vi "Frequency Response Function (Mag-Phase) 1-N.vi"(0 "time signal X":waveform(dbl), 1 "restart averaging (F)":bool, 2 "window parameter":dbl=nan, 5 "time signals Y":waveform(dbl)[](array[waveform]), 7 "window":T1=1 items=["Rectangle"=0, "Hanning"=1, "Hamming"=2, "Blackman-Harris"=3, "Exact Blackman"=4, "Blackman"=5, "Flat Top"=6, "4 Term B-Harris "=7, "7 Term B-Harris"=8, "Low Sidelobe"=9, "Blackman Nuttall"=11, "Triangle"=30, "Bartlett-Hanning"=31, "Bohman"=32, "Parzen"=33, "Welch"=34, "Kaiser"=60, "Dolph-Chebyshev"=61, "Gaussian"=62], 9 "view":T3, 11 "error in (no error)":errorcluster, 12 "averaging parameters":T2={"averaging mode"=enum."No averaging", "weighting mode"=enum."Exponential", "number of averages"=10} {"number of averages" min=1}, 13 "FRF Mode":enum16{"H1", "H2", "H3"}(ring)) -> (3 "averaging done":bool, 4 "magnitudes":cluster{"f0":dbl, "df":dbl, "magnitude":dbl[]}[](array[cluster]) {"magnitude" format="%.2p"; "f0" format="%0.2p"; "df" format="%0.2p"}, 6 "phases":cluster{"f0":dbl, "df":dbl, "phase":dbl[]}[](array[cluster]) {"phase" format="%.2p"; "f0" format="%0.2p"; "df" format="%0.2p"}, 8 "coherences":cluster{"f0":dbl, "df":dbl, "coherence":dbl[]}[](array[cluster]), 10 "averages completed":dbl format="%.2p", 15 "error out":errorcluster)   [LabVIEW 2020, in "NI_MAPro.lvlib"]
doc: "Computes the frequency response and the coherence based on the input signals. Results are returned as <B>magnitude</B>, <B>phase</B>, and <B>coherence</B>."
uses:
  NI_MAPro.lvlib
  windowTd.ctl
  2-chan State.ctl
  NI_MABase.lvlib
  NI_AALPro.lvlib
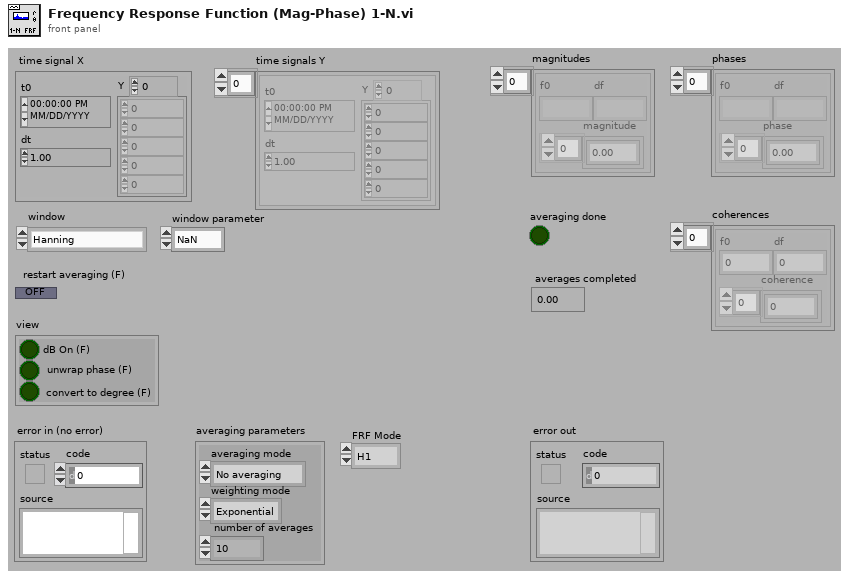
[diagram p1: front panel]
types:
  T1 = typedef "NI_AALPro.lvlib/windowTd.ctl" = u32
  T2 = cluster{"averaging mode":enum16{"No averaging", "Vector averaging", "RMS averaging", "Peak hold"}, "weighting mode":enum16{"Linear", "Exponential"}, "number of averages":u32}
  T3 = cluster{"dB On (F)":bool, "unwrap phase (F)":bool, "convert to degree (F)":bool}
  T4 = typedef "NI_MAPro.lvlib/2-chan State.ctl" = cluster{"Sx":cdb[], "Sy":cdb[], "Sxx":dbl[], "Syy":dbl[], "Sxy":cdb[], "block size":i32, "df":dbl, "dt":dbl, "avgs completed":dbl, "spectrum parameters":cluster{"averaging parameters":cluster{"averaging mode":enum16{"No averaging", "Vector averaging", "RMS averaging", "Peak hold"}, "weighting mode":enum16{"Linear", "Exponential"}, "number of averages":u32}, "window":T1}, "lin avg done":bool, "t0 history":dbl, "dt history":dbl, "timestamp":dbl}
  T5 = cluster{"f0":dbl, "df":dbl, "imag or phase":dbl[]}
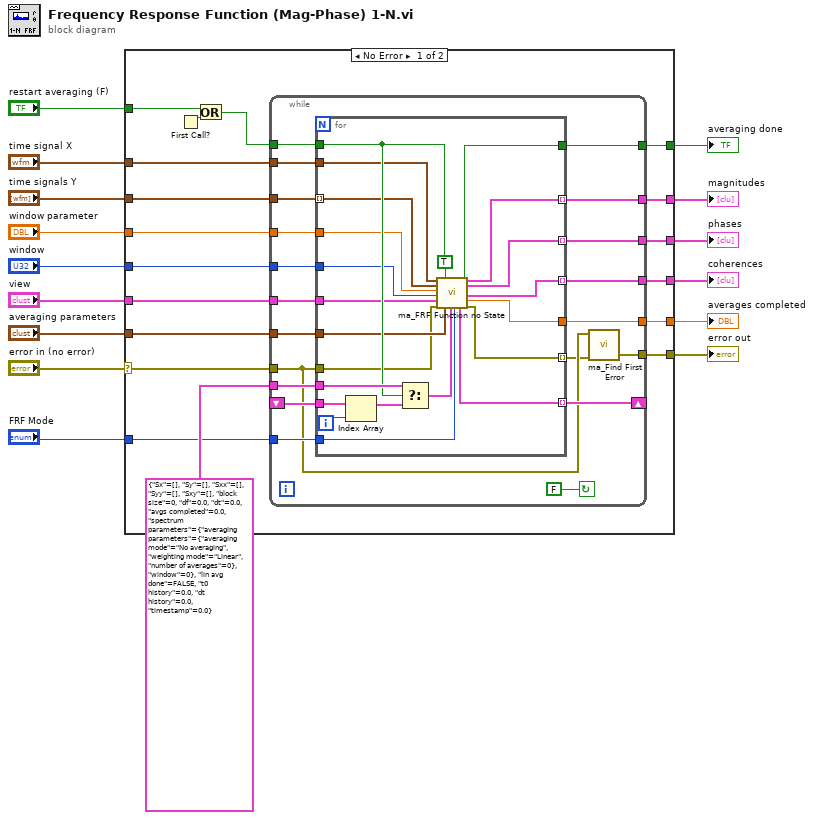
[diagram p0: block diagram]
diagram:
  n1 = case shown="No Error" "error in (no error)" {
    selector: "error in (no error)" -> [w30 w76]
    tunnel: [w29 w76] -> w14
    tunnel: "FRF Mode" -> [w28 _]
    tunnel: "averaging parameters" -> [w27 _]
    tunnel: "view" -> [w26 _]
    tunnel: "window" -> [w25 _]
    tunnel: "time signals Y" -> [w24 _]
    tunnel: "time signal X" -> [w23 _]
    tunnel: "restart averaging (F)" -> [w22 _]
    tunnel: "window parameter" -> [w21 _]
    tunnel: [w20 _] -> w5
    tunnel: [w19 _] -> w4
    tunnel: [w18 _] -> w3
    tunnel: [w17 _] -> w2
    tunnel: [w16 _] -> w1
    frame No Error {
      n2 = First Call?() -> (First Call?: T/F=w33:bool)
      n3 = Or(x=w22, y=w33) -> (x .or. y?=w31:bool)
      n4 = while {
        tunnel: T4 {"Sx"=[], "Sy"=[], "Sxx"=[], "Syy"=[], "Sxy"=[], "block size"=0, "df"=0.0, "dt"=0.0, "avgs completed"=0.0, "spectrum parameters"={"averaging parameters"={"averaging mode"=enum."No averaging", "weighting mode"=enum."Linear", "number of averages"=0}, "window"=0}, "lin avg done"=FALSE, "t0 history"=0.0, "dt history"=0.0, "timestamp"=0.0} ("state info out") -> [w53]
        tunnel: w31 -> [w52]
        tunnel: w23 -> [w51]
        tunnel: w24 -> [w50]
        tunnel: w25 -> [w49]
        tunnel: w26 -> [w48]
        tunnel: w27 -> [w47]
        tunnel: w28 -> [w46]
        tunnel: [w45] -> w20
        tunnel: [w44] -> w16
        tunnel: w30 -> [w37]
        tunnel: [w43] -> w19
        tunnel: [w42] -> w18
        tunnel: [w41] -> w17
        shift-right: [w39] -> _
        shift-left: _ -> [w38]
        tunnel: [w35] -> w29
        tunnel: w21 -> [w34]
        stop <- FALSE continue-if-true
        n5 = for {
          tunnel: w52 -> [w68]
          tunnel: [w75] -> w45
          tunnel: [w74] -> w44
          tunnel: [w73] -> w43 mode=indexing
          tunnel: [w70] -> w42 mode=indexing
          tunnel: w53 -> [w69]
          tunnel: w51 -> [w67]
          tunnel: w50 -> [w60] mode=indexing
          tunnel: w49 -> [w66]
          tunnel: w48 -> [w65]
          tunnel: w47 -> [w64]
          tunnel: w46 -> [w63]
          tunnel: [w62] -> w41 mode=indexing
          tunnel: w37 -> [w61]
          tunnel: [w59] -> w39 mode=indexing
          tunnel: w38 -> [w57]
          tunnel: [w55] -> w36 mode=indexing
          tunnel: w34 -> [w54]
          i -> [w58]
          n6 = Index Array(array=w57, index=w58) -> (element=w56:T4)
          n7 = Select(t=w69, s=w68, f=w56) -> (s? t:f=w72:T4)
          n8 = call "ma_FRF Function no State.vi"("time signal X"=w67, "time signal Y"=w60, "window parameter"=w54, "window"=w66, "view"=w65, "error in (no error)"=w61, "restart averaging (F)"=w68, "averaging parameters"=w64, "mag-phase"=TRUE, "state info"=w72, "FRF Mode"=w63) -> ("averaging done"=w75:bool, "state info out"=w59:T4, "real or mag"=w73:cluster{"f0":dbl, "df":dbl, "real or mag":dbl[]}, "imag or phase"=w70:T5, "coherence"=w62:cluster{"f0":dbl, "df":dbl, "coherence":dbl[]}, "averages completed"=w74:dbl, "error out"=w55:errorcluster)  [unwired: 2 out]
        }
        n9 = call "ma_Find First Error.vi"("error array in"=w36, "error in 1 (no error)"=w37) -> ("error out"=w35:errorcluster)  [unwired: 2 in, 3 out]
      }
    }
    frame Error {
    }
  }
  "error out" <- w14
  "averages completed" <- w1
  "averaging done" <- w5
  "coherences" <- w2
  "magnitudes" <- w4
  "phases" <- w3
